vi "Add Labels.vi"(8 "error in":errorcluster, 10 "labels":T2[](array[typedef]) {"Label (octal)" format="%o"}, 11 "port ref":T1 format="%.0x") -> (0 "error out":errorcluster, 3 "port ref out":T1 format="%.0x")   [LabVIEW 2020, in "Ballard ARINC 429 Scripting.lvlib"]
uses:
  Ballard ARINC 429 Scripting.lvlib
  <vilib>/NI VeriStand/Custom Device API/Custom Device Item Ref.ctl
  Import/Types/Label.ctl
  Import/Types/Parameter.ctl
  Encoding and Decoding/Encoding.ctl
  Shared/Label Properties.ctl
  <vilib>/NI VeriStand/Custom Device API/Custom Device API.lvlib
  Encoding and Decoding/Encoding and Decoding.lvlib
  Import/ARINC 429 Import.lvlib
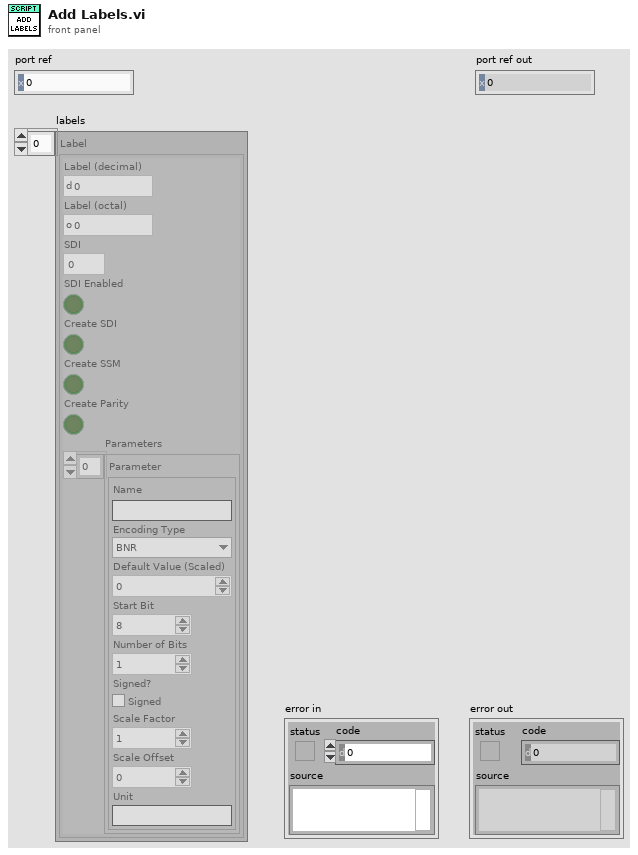
[diagram p1: front panel]
types:
  T1 = typedef "Custom Device API.lvlib/Custom Device Item Ref.ctl" = u64
  T2 = typedef "ARINC 429 Import.lvlib/Label.ctl" = cluster{"Label (decimal)":i32, "Label (octal)":i32, "SDI":u8, "SDI Enabled":bool, "Create SDI":bool, "Create SSM":bool, "Create Parity":bool, "Parameters":T3[]}
  T3 = typedef "ARINC 429 Import.lvlib/Parameter.ctl" = cluster{"Name":string, "Encoding Type":T4, "Default Value (Scaled)":dbl, "Start Bit":i32, "Number of Bits":i32, "Signed?":bool, "Scale Factor":dbl, "Scale Offset":dbl, "Unit":string}
  T4 = typedef "Encoding and Decoding.lvlib/Encoding.ctl" = enum16{"BNR", "BCD", "Discrete"}
  T5 = typedef "Label Properties.ctl" = cluster{"label (Dec)":i32, "SDI value":u8, "SDI enabled":bool}
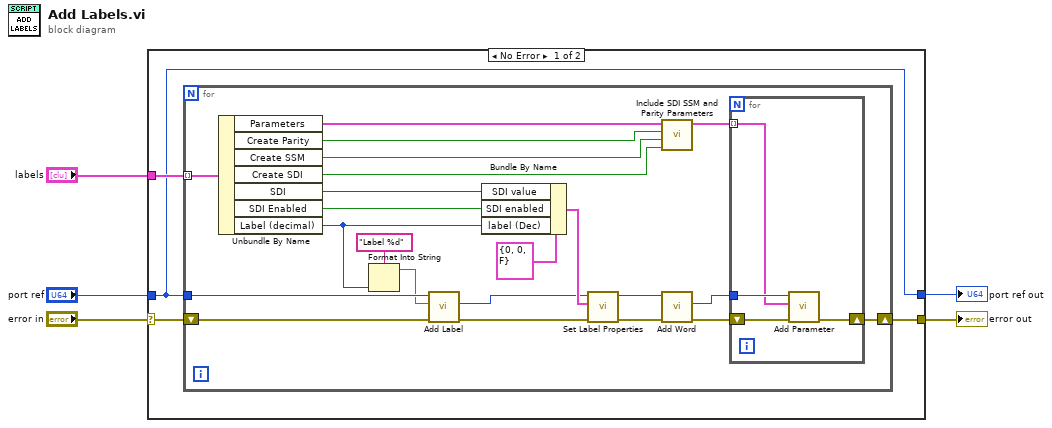
[diagram p0: block diagram]
diagram:
  n1 = case shown="No Error" "error in" {
    selector: "error in" -> [w9 w37]
    tunnel: "port ref" -> [w6 w36]
    tunnel: [w8 w37] -> w4
    tunnel: "labels" -> [w7 _]
    tunnel: [w6 w36] -> w1
    frame No Error {
      n2 = for {
        tunnel: w7 -> [w31] mode=indexing
        shift-right: [w20] -> w8
        shift-left: w9 -> [w30]
        tunnel: w6 -> [w29]
        n3 = Unbundle By Name(w31) -> ("Parameters"=w15:T3[], "Create Parity"=w14:bool, "Create SSM"=w13:bool, "Create SDI"=w12:bool, "SDI"=w21:u8, "SDI Enabled"=w22:bool, "Label (decimal)"=w23:i32)
        n4 = Format Into String(format string="Label %d", w23) -> (resulting string=w27:string)  [unwired: 2 in, 1 out]
        n5 = call "Add Label.vi"("error in"=w30, "name"=w27, "port ref"=w29) -> ("error out"=w26:errorcluster, "label ref"=w11:T1)  [unwired: 5 in, 2 out]
        n6 = Bundle By Name(cluster=T5 {"label (Dec)"=0, "SDI value"=0, "SDI enabled"=FALSE} ("label properties"), "SDI value"=w21, "SDI enabled"=w22, "label (Dec)"=w23) -> (w25:T5)
        n7 = call "Set Label Properties.vi"("error in"=w26, "label properties"=w25, "label ref"=w11) -> ("error out"=w19:errorcluster, "label ref out"=w17:T1)  [unwired: 7 in]
        n8 = call "Include SDI SSM and Parity Parameters.vi"("create SDI (F)"=w12, "create SSM (F)"=w13, "create parity (F)"=w14, "parameters"=w15) -> ("parameters out"=w16:T3[])  [unwired: 7 in]
        n9 = call "Add Word.vi"("error in"=w19, "label ref"=w17) -> ("error out"=w18:errorcluster, "word ref"=w10:T1)  [unwired: 6 in, 2 out]
        n10 = for {
          shift-right: [w33] -> w20
          shift-left: w18 -> [w34]
          tunnel: w16 -> [w32] mode=indexing
          tunnel: w10 -> [w35]
          n11 = call "Add Parameter.vi"("error in"=w34, "parameter"=w32, "word ref"=w35) -> ("error out"=w33:errorcluster)  [unwired: 6 in, 2 out]
        }
      }
    }
    frame Error {
    }
  }
  "error out" <- w4
  "port ref out" <- w1
